vi "Control - Generic - Spark Host.vi"() -> ()   [LabVIEW 2015, in "ECS-Host.lvlib"]
uses:
  ECS-Host.lvlib
  <vilib>/addons/Software Calibration Management/XControls/TBL1D.xctl
  <vilib>/addons/Software Calibration Management/XControls/TBL2D.xctl
panel:
  in  "SparkAdv_Man":sgl[](array[numeric]) caption="[DBTDC]"
  in  "MaxEngineSpeed":sgl caption="[RPM]"
  out "RampKickAdv_Des":sgl[](array[numeric]) caption="[CAD]"
  out "Knock":u8 caption="[]"
  out "_Knock":bool[](array[boolean]) caption="Knock"
  out "MainDwell_TblOut":sgl caption="[ms]"
  in  "NextCycleSparkAdv_E":bool caption="Enable Inj"
  out "NextCycleSparkAdvAvg":sgl caption="[CAD]"
  out "SparkDwell_Des":sgl[](array[numeric]) caption="[ms]"
  out "_Pulse Gen Labels":string[](array[string]) caption="[]"
  out "SparkAdv_Des":sgl[](array[numeric]) caption="[DBTDC]"
  in  "MainDwell_Man":sgl caption="[ms]"
  in  "MainDwell_ManE":bool caption="Enable Inj"
  out "SparkAdv_TblOut":sgl caption="[CAD]"
  out "SparkAdvWarmup_TblOut":sgl caption="[CAD]"
  out "SparkAdvBoost_TblOut":sgl caption="[CAD]"
  out "SparkAdvEGR_TblOut":sgl caption="[CAD]"
  out "SparkAdv_Calc":sgl caption="[CAD]"
  in  "EngineOverspeedSparkRet":sgl caption="[CAD]"
  in  "SparkAdv_ManE":bool caption="Enable Inj"
  in  "_Spark Timing Table":T1(tab) caption="_Spark Tab Control"
  in  "SparkAdv_Tbl":cluster{"X":sgl[], "Y":sgl[], "Z":sgl[][]}(xcontrol) caption="[]"
  in  "SparkAdvWarmup_Tbl":cluster{"X":sgl[], "Y":sgl[]}(xcontrol) caption="[]"
  in  "SparkAdvBoost_Tbl":cluster{"X":sgl[], "Y":sgl[]}(xcontrol) caption="[]"
  in  "SparkAdvBoost_E":bool caption="Enable Inj"
  in  "SparkAdvEGR_Tbl":cluster{"X":sgl[], "Y":sgl[]}(xcontrol) caption="[]"
  in  "SparkAdvEGR_E":bool caption="Enable Inj"
  in  "SparkAdvRampKick_E":bool caption="Enable Inj"
  in  "ReKickDelay":sgl caption="[s]"
  in  "KickMagnitude":sgl caption="[CAD]"
  in  "RampKickGain":sgl caption="[CAD/s]"
  in  "RampKickMin":sgl caption="[CAD]"
  in  "RampKickMax":sgl caption="[CAD]"
  in  "MainDwell_Tbl":cluster{"X":sgl[], "Y":sgl[]}(xcontrol) caption="[]"
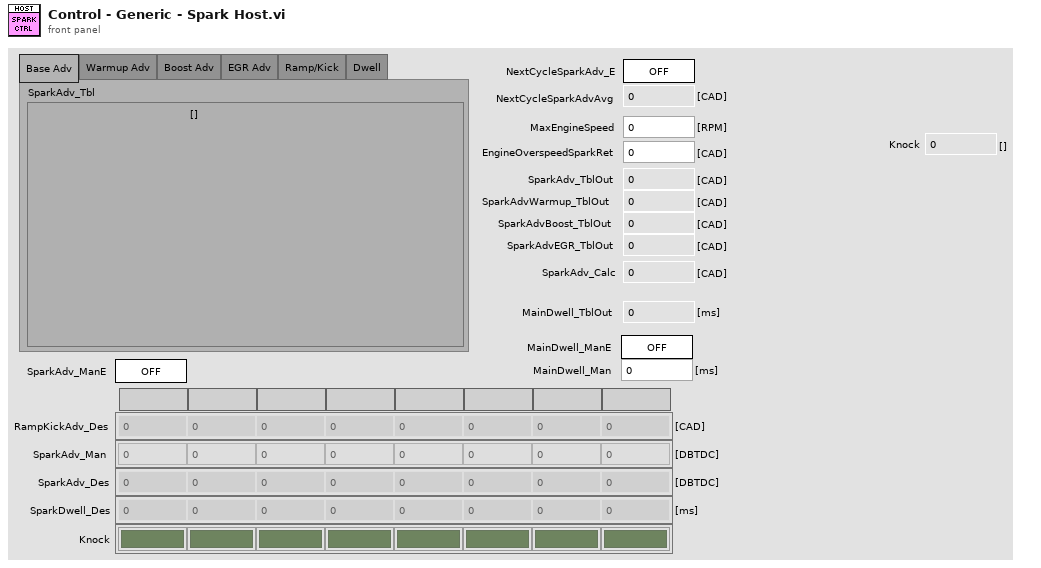
[diagram p1: front panel]
types:
  T1 = enum32{"Base Adv", "Warmup Adv", "Boost Adv", "EGR Adv", "Ramp/Kick", "Dwell"}
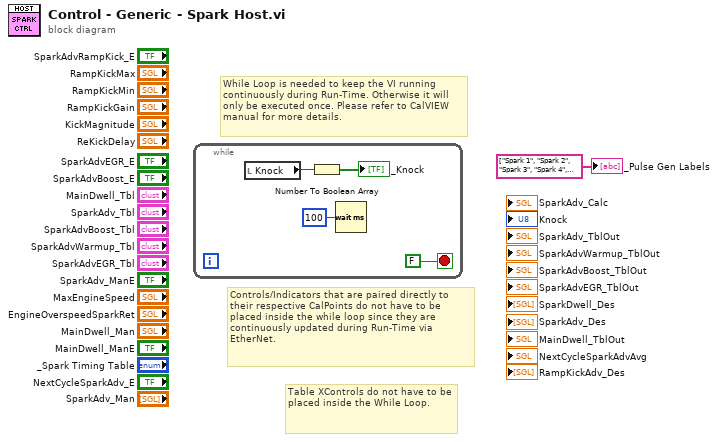
[diagram p0: block diagram]
diagram:
  # "Table XControls do not have to be placed inside the While Loop."
  # "While Loop is needed to keep the VI running\ncontinuously during Run-Time. Otherwise it will only be executed once. Please refer to CalVIEW manual for more details."
  # "Controls/Indicators that are paired directly to their respective CalPoints do not have to be placed inside the while loop since they are continuously updated during Run-Time via EtherNet."
  n1 = while {
    stop <- FALSE stop-if-true
    n2 = local read "Knock"() -> (w3:u8)
    n3 = Number To Boolean Array(number=w3) -> (Boolean array=→"_Knock":bool[])
    n4 = Wait (ms)(milliseconds to wait=u32 100 ("millisecondstowait")) -> ()  [unwired: 1 out]
  }
  "_Pulse Gen Labels" <- string[] ["Spark 1", "Spark 2", "Spark 3", "Spark 4", "Spark 5", "Spark 6", "Spark 7", "Spark 8"] ("_Pulse Gen Labels")
